vi "setTrigger.vi"(8 "error in (no error)":errorcluster, 9 "Args":string[](array[string]), 10 "Command":string, 11 "TektronixDPOSimple in":refnum<class "RohdeSchwarz_RTA4000.lvclass">) -> (0 "error out":errorcluster, 2 "new commands":string, 3 "TektronixDPOSimple out":refnum<class "RohdeSchwarz_RTA4000.lvclass">)   [LabVIEW 2020, in "RohdeSchwarz_RTA4000.lvclass"]
doc: "Set the speficied Trigger subproperty value, and update the CVT"
uses:
  RohdeSchwarz_RTA4000.lvclass
  Tektronix DPO MSO 2000 4000 Series/Tektronix DPO MSO 2000 4000 Series.lvlib
  Tektronix DPO MSO 2000 4000 Series/Public/Configure/Configure Trigger (Edge).vi
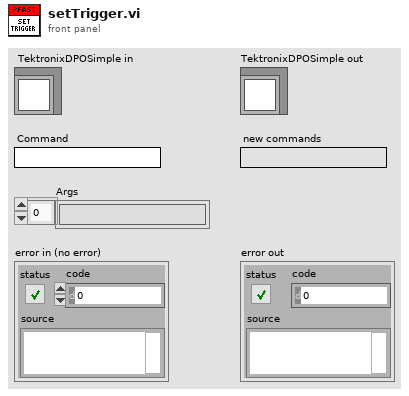
[diagram p1: front panel]
types:
  T1 = typedef "TriggerModes.ctl" = u16
  T2 = typedef "TriggerCluster.ctl" = cluster{"Mode":T1, "Source":u16, "Coupling":u16, "Level":dbl, "Slope":u16}
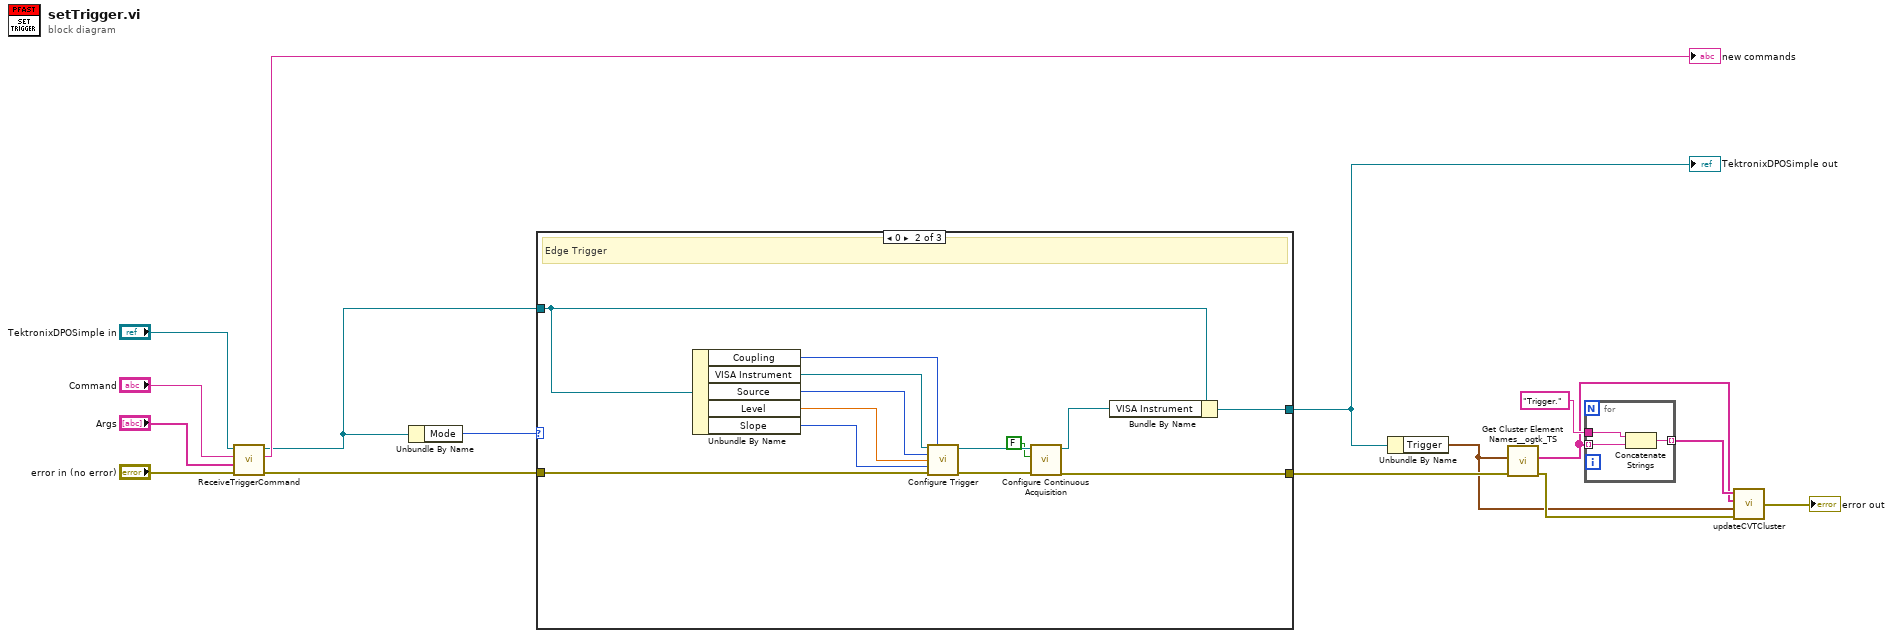
[diagram p0: block diagram]
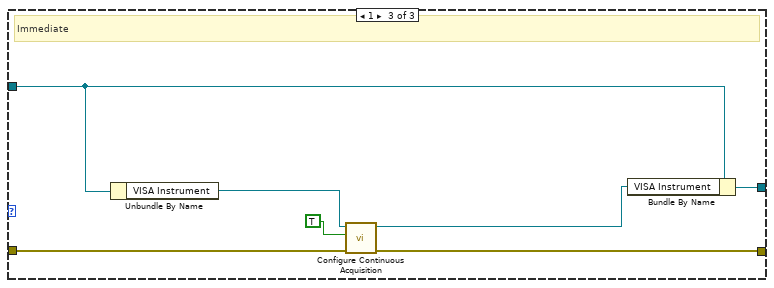
[diagram p3: hidden frame]
diagram:
  n1 = call "ReceiveTriggerCommand.vi"("error in (no error)"="error in (no error)", "Args"="Args", "Command"="Command", "TektronixDPOSimple in"="TektronixDPOSimple in") -> ("error out"=w6:errorcluster, "new commands"=→"new commands":string, "TektronixDPOSimple out"=w4:refnum<class "RohdeSchwarz_RTA4000.lvclass">)  [unwired: 5 in]
  n2 = Unbundle By Name(w4) -> ("Mode"=w7:T1)
  n3 = case shown="0" w7 {
    tunnel: w6 -> [w18 w31 w37]
    tunnel: [w18 w22 w32] -> w5
    tunnel: w4 -> [w17 w25 w35]
    tunnel: [w17 w24 w34] -> w3
    frame Default {
    }
    frame 0 {
      # "Edge Trigger"
      n4 = Unbundle By Name(w25) -> ("Coupling"=w30:u16, "VISA Instrument"=w29:refnum<visa-resource-name>, "Source"=w28:u16, "Level"=w27:dbl, "Slope"=w26:u16)
      n5 = call-poly "Configure Trigger.vi"("VISA resource name"=w29, "Trigger Coupling (0 : DC)"=w30, "Trigger Source (0: Channel 1)"=w28, "Trigger Level (0.0 V)"=w27, "Trigger Slope (0: Rising)"=w26, "error in (no error)"=w31) -> ("VISA resource name out"=w21:refnum<visa-resource-name>, "error out"=w23:errorcluster)  [unwired: 8 in]
      n6 = call "Configure Continuous Acquisition.vi"("error in (no error)"=w23, "Enable Continuous Acquisition Mode (T: Enable)"=FALSE, "VISA resource name"=w21) -> ("error out"=w22:errorcluster, "VISA resource name out"=w19:refnum<visa-resource-name>)  [unwired: 7 in]
      n7 = Bundle By Name(cluster=w25, "VISA Instrument"=w19) -> (w24:refnum<class "RohdeSchwarz_RTA4000.lvclass">)
    }
    frame 1 {
      # "Immediate"
      n8 = Unbundle By Name(w35) -> ("VISA Instrument"=w36:refnum<visa-resource-name>)
      n9 = call "Configure Continuous Acquisition.vi"("error in (no error)"=w37, "Enable Continuous Acquisition Mode (T: Enable)"=TRUE, "VISA resource name"=w36) -> ("error out"=w32:errorcluster, "VISA resource name out"=w33:refnum<visa-resource-name>)  [unwired: 7 in]
      n10 = Bundle By Name(cluster=w35, "VISA Instrument"=w33) -> (w34:refnum<class "RohdeSchwarz_RTA4000.lvclass">)
    }
  }
  "TektronixDPOSimple out" <- w3
  n11 = Unbundle By Name(w3) -> ("Trigger"=w1:T2)
  n12 = call "Get Cluster Element Names__ogtk_TS.vi"("error in (no error)"=w5, "Variant"=w1) -> ("error out"=w2:errorcluster, "Names (Array)"=w14:string[])  [unwired: 8 in]
  n13 = for {
    tunnel: w14 -> [w41] mode=indexing
    tunnel: "Trigger." -> [w40]
    tunnel: [w39] -> w16 mode=indexing
    n14 = Concatenate Strings(w40, w41) -> (w39:string)
  }
  n15 = call "updateCVTCluster.vi"("error in"=w2, "variant (destination) out"=w1, "Cluster Names"=w14, "CVT Names"=w16) -> ("error out"=→"error out":errorcluster)
